vi "ElapsedSecs.vi"(8 "error in (no error)":errorcluster, 11 "Function":T1(ring)) -> (0 "error out":errorcluster, 1 "Elapsed msecs since last check":u32, 2 "ElapsedTime":string, 3 "Elapsed secs since start":i32, 4 "Start Time":string, 5 "Start Date":string, 6 "Elapsed mm:ss":string)   [LabVIEW 2013]
uses:
  Main Support/Global 2.vi
panel:
  in  "Start Time":timestamp
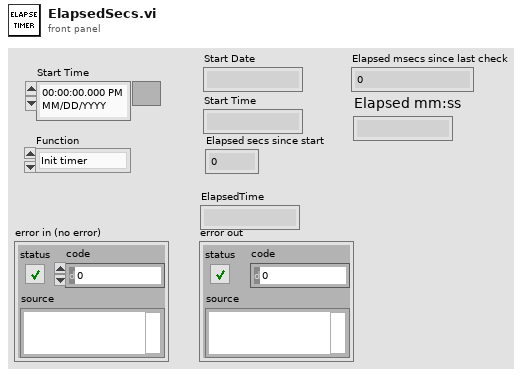
[diagram p1: front panel]
types:
  T1 = enum16{"Init timer", "Get elapsed time (msec)", "Stop timer"}
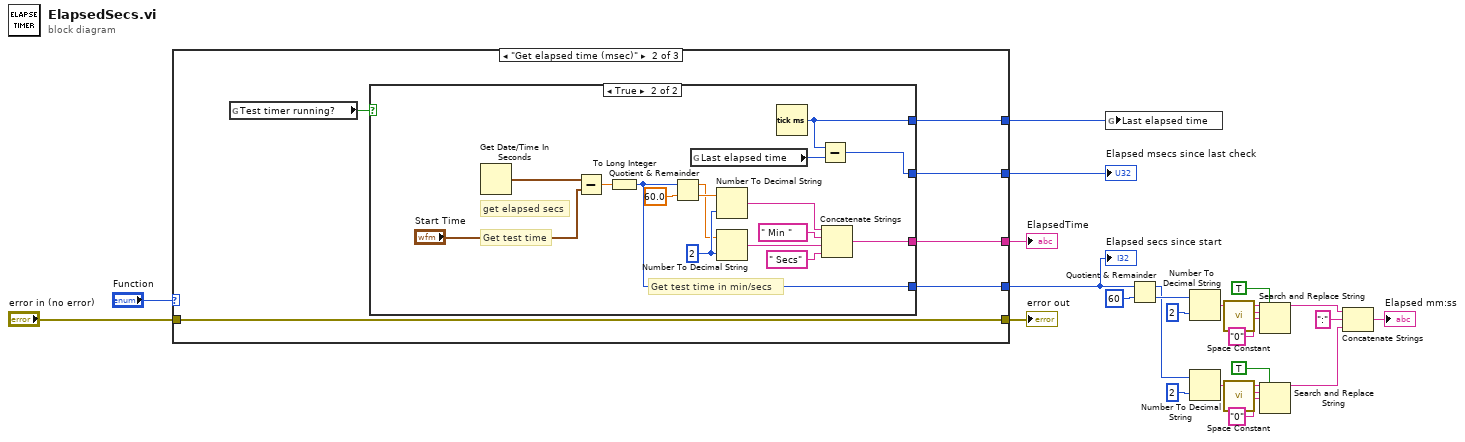
[diagram p0: block diagram]
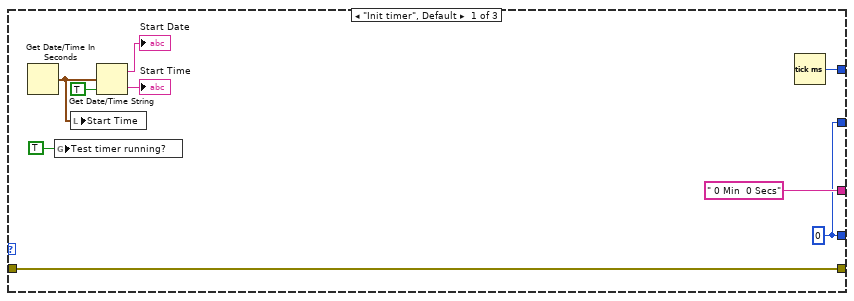
[diagram p2: hidden frame]
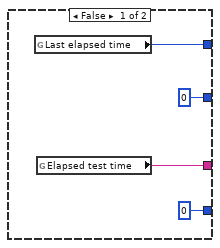
[diagram p3: hidden frame]
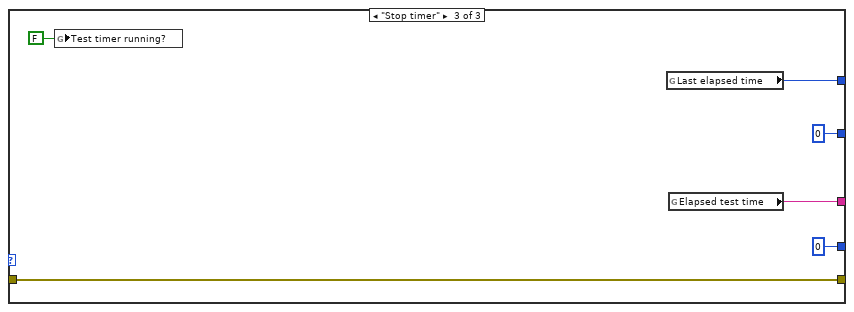
[diagram p4: hidden frame]
diagram:
  n1 = case shown="\"Get elapsed time (msec)\"" "Function" {
    tunnel: [w31 w39 w65] -> w23
    tunnel: "error in (no error)" -> [w31 w39 w65]
    tunnel: [" 0 Min  0 Secs" w38 w63] -> w21
    tunnel: [w26 w37 0] -> w18
    tunnel: [w26 w36 u32 0] -> w20
    tunnel: [w27 w35 w62] -> w19
    frame "Init timer", Default {
      w26 = 0
      n2 = Get Date/Time In Seconds() -> (seconds since 1Jan1904=w28:timestamp)
      n3 = global write "Global 2.vi" "Test timer running?"(TRUE ("Test timer running?")) -> ()
      n4 = local write "Start Time"(w28) -> ()
      n5 = Get Date/Time String(seconds (now)=w28, want seconds? (F)=TRUE) -> (date string=→"Start Date":string, time string=→"Start Time":string)  [unwired: 1 in]
      n6 = Tick Count (ms)() -> (millisecond timer value=w27:u32)
    }
    frame "Get elapsed time (msec)" {
      n7 = global read "Global 2.vi" "Test timer running?"() -> (w34:bool)
      n8 = case shown="True" w34 {
        tunnel: [w41 w49] -> w38
        tunnel: [0 w47] -> w37
        tunnel: [u32 0 w45] -> w36
        tunnel: [w43 w44] -> w35
        frame False {
          n9 = global read "Global 2.vi" "Last elapsed time"() -> (w43:u32)
          n10 = global read "Global 2.vi" "Elapsed test time"() -> (w41:string)
        }
        frame True {
          w56 = i16 2 ("width (-)")
          # "Get test time"
          # "Get test time in min/secs"
          # "get elapsed secs"
          n11 = Get Date/Time In Seconds() -> (seconds since 1Jan1904=w59:timestamp)
          n12 = Subtract(x=w59, y="Start Time") -> (x-y=w58:dbl)
          n13 = To Long Integer(number=w58) -> (32bit integer=w47:i32)
          n14 = Quotient & Remainder(x=w47, y=60.0) -> (x-y*floor(x/y)=w54:dbl, floor(x/y)=w55:dbl)
          n15 = global read "Global 2.vi" "Last elapsed time"() -> (w46:u32)
          n16 = Number To Decimal String(number=w55, width (-)=w56) -> (decimal integer string=w50:string)
          n17 = Number To Decimal String(number=w54, width (-)=w56) -> (decimal integer string=w52:string)
          n18 = Tick Count (ms)() -> (millisecond timer value=w44:u32)
          n19 = Subtract(x=w44, y=w46) -> (x-y=w45:u32)
          n20 = Concatenate Strings(w50, " Min " ("string"), w52, " Secs" ("string")) -> (w49:string)
        }
      }
    }
    frame "Stop timer" {
      n21 = global write "Global 2.vi" "Test timer running?"(FALSE ("Test timer running?")) -> ()
      n22 = global read "Global 2.vi" "Last elapsed time"() -> (w62:u32)
      n23 = global read "Global 2.vi" "Elapsed test time"() -> (w63:string)
    }
  }
  "error out" <- w23
  "ElapsedTime" <- w21
  "Elapsed secs since start" <- w18
  "Elapsed msecs since last check" <- w20
  n24 = global write "Global 2.vi" "Last elapsed time"(w19) -> ()
  n25 = Quotient & Remainder(x=w18, y=60) -> (x-y*floor(x/y)=w13:i32, floor(x/y)=w16:i32)
  n26 = Number To Decimal String(number=w16, width (-)=i16 2) -> (decimal integer string=w10:string)
  n27 = Number To Decimal String(number=w13, width (-)=i16 2) -> (decimal integer string=w3:string)
  n28 = call <vilib>:"Space Constant.vi"() -> ("String"=w9:string)
  n29 = call <vilib>:"Space Constant.vi"() -> ("String"=w4:string)
  n30 = Search and Replace String(replace all?=TRUE ("replace all? (F)"), input string=w10, search string=w9, replace string="0" ("replace string (\"\")")) -> (result string=w6:string)  [unwired: 4 in, 3 out]
  n31 = Search and Replace String(replace all?=TRUE ("replace all? (F)"), input string=w3, search string=w4, replace string="0" ("replace string (\"\")")) -> (result string=w1:string)  [unwired: 4 in, 3 out]
  n32 = Concatenate Strings(w6, ":" ("string"), w1) -> (→"Elapsed mm:ss":string)
